vi "Chain4.vi"(7 "Name (\"\" to Use UUID)":string="CSM-Module") -> ()   [LabVIEW 2017, in "CSM-Testcase.lvlib"]
doc: "Creates a template for a CSM module without a user interface.\n\n> [!NOTE] CSM Name Rules\n> - The CSM module name must be unique to avoid entering the \"Critical Error\" state.\n> - If the input is \"\", a UUID will be used as the module name. This module will operate in independent mode and will not be listed in the module list.\n> - If the input ends with '#', the module will run in work mode. Modules with the same name will share the same message queue. External messages will be handled by the idle module.\n\n> [!NOTE] CSM Initialization State\n> - The default value is \"Macro: Initialize\", consistent with the JKISM state machine.\n> - This state is typically not modified and is provided to facilitate external programmatic changes to the initialization state.\n\n\n-- <b>Controls</b> --\n- <b>Name (\"\" to Use UUID)</b>: CSM Module Name\n- <b>Init State(\"Macro: Initialize\")</b>: Initialization State, default is \"Macro: Initialize\""
uses:
  CSM-Testcase.lvlib
  src/user.lib/_NEVSTOP/Communicable State Machine(CSM)/AdvanceAPI/CSM - Revert Arguments-Safe String.vi
  src/user.lib/_NEVSTOP/Communicable State Machine(CSM)/AdvanceAPI/CSM - Make String Arguments Safe.vi
  src/user.lib/_NEVSTOP/Communicable State Machine(CSM)/AdvanceAPI/CSM - Break Down Multiple States String.vi
  src/user.lib/_NEVSTOP/Communicable State Machine(CSM)/AdvanceAPI/CSM - Keywords.vi
  src/user.lib/_NEVSTOP/Communicable State Machine(CSM)/_Shared/Trim Single-line Text.vi
  Global-TestcaseCSM.vi
  src/user.lib/_NEVSTOP/Communicable State Machine(CSM)/_Polymophic/Build No-Reply Asynchronous Message with Arguments.vi
  src/user.lib/_NEVSTOP/Communicable State Machine(CSM)/_Polymophic/Build Asynchronous Message with Arguments.vi
  src/user.lib/_NEVSTOP/Communicable State Machine(CSM)/_Polymophic/Build Register Message.vi
  src/user.lib/_NEVSTOP/Communicable State Machine(CSM)/_Polymophic/Build Interrupt Broadcast Message.vi
  src/user.lib/_NEVSTOP/Communicable State Machine(CSM)/Communicable State Machine.lvlib
panel:
  out "Error Occurred":errorcluster
  out "State History":string
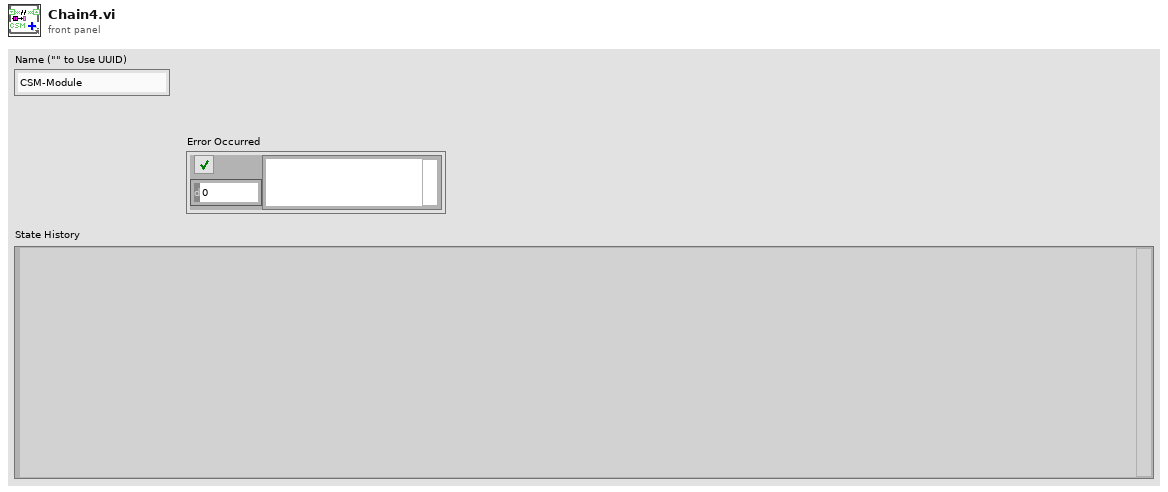
[diagram p1: front panel]
types:
  T1 = cluster{"Arguments":string, "Response":string, "error":errorcluster}
  T2 = enum32{"Invalid", "Standard", "Closed", "Hidden", "Minimized", "Maximized"}
  T3 = enum32{"invalid app kind", "Development System", "Run Time System", "Student Edition", "Embedded LabVIEW", "Evaluation", "Custom"}
  T4 = typedef "Communicable State Machine.lvlib/_CSM_Response Source Message.ctl" = cluster{"‘State":string, "’Arguments":string, "’Error":errorcluster}
  T5 = cluster{"Current VI Reference":refnum<vi>, "Close Panel on Exit?":bool}
  T6 = cluster{"Core":cluster{"Current VI Reference":refnum<vi>, "Close Panel on Exit?":bool}, "Your Boolean data":bool, "Your string data":string, "Counter":u32}
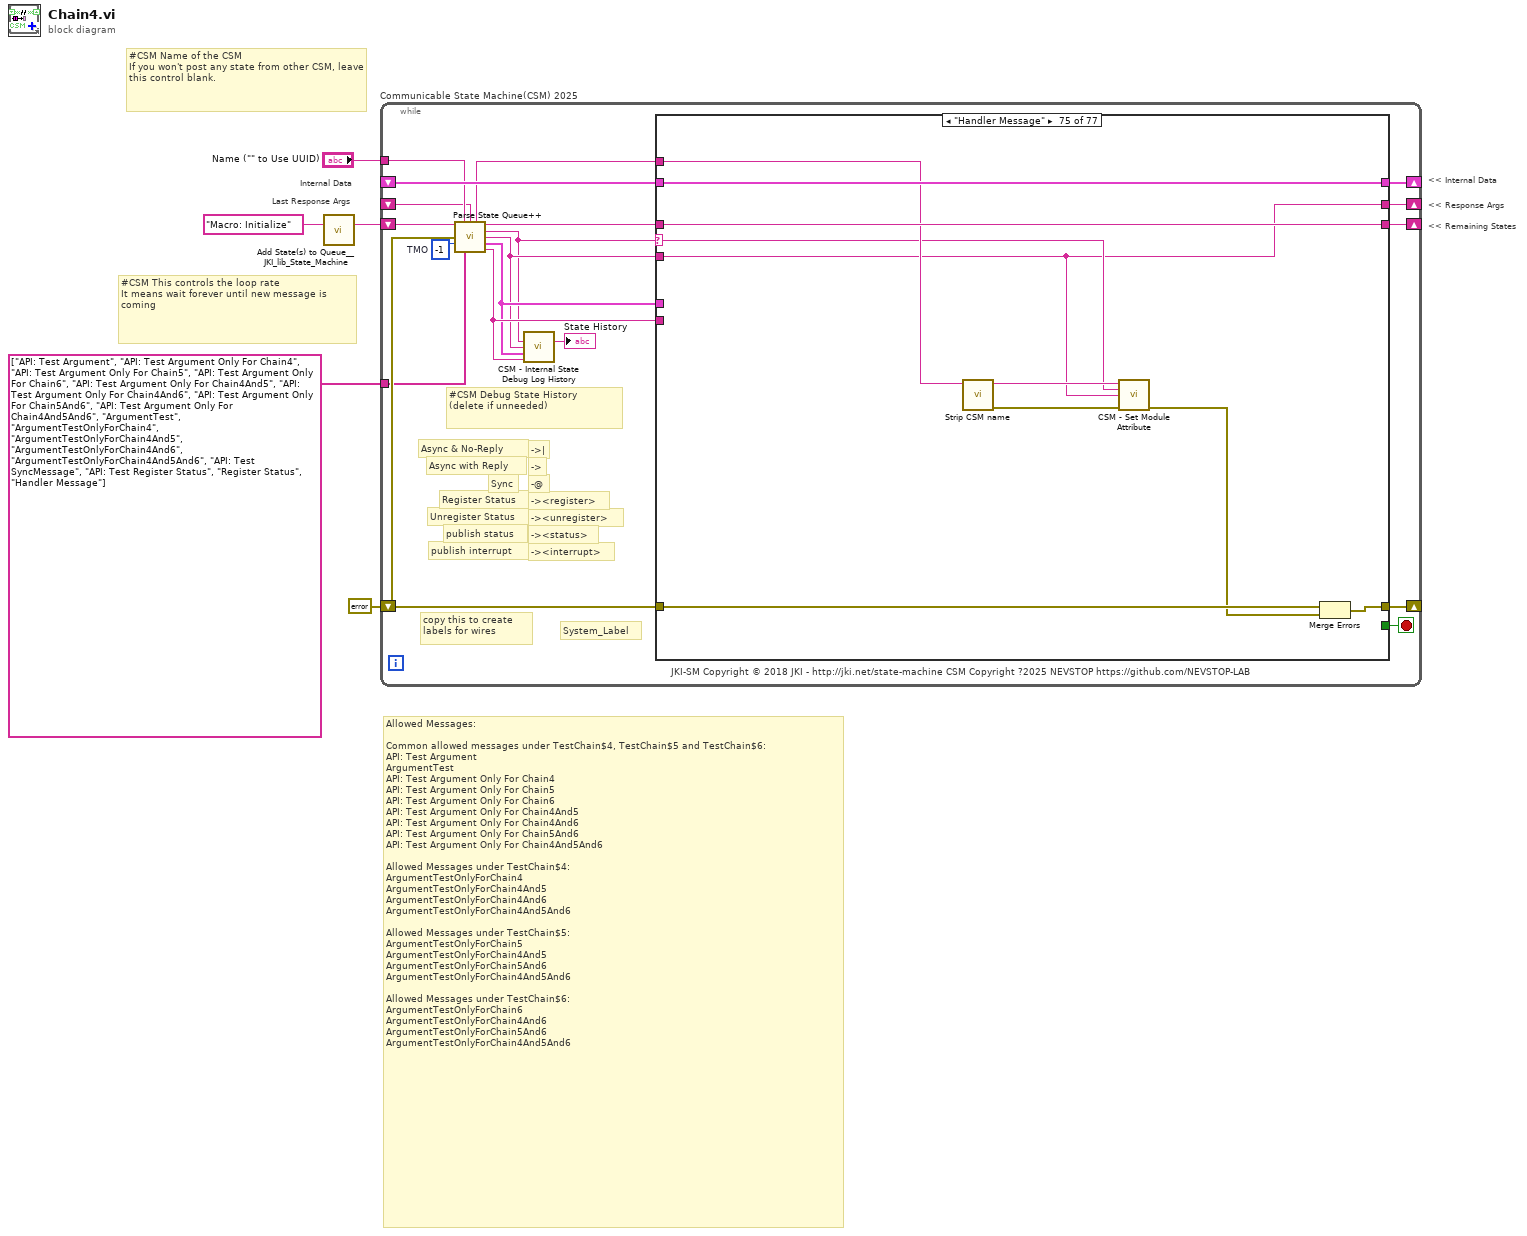
[diagram p0: block diagram]
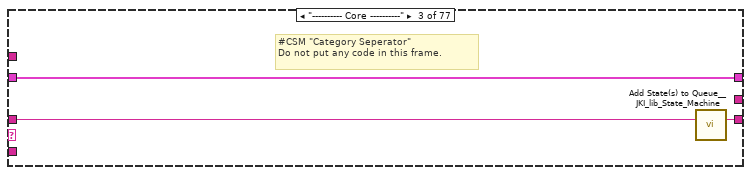
[diagram p4: hidden frame]
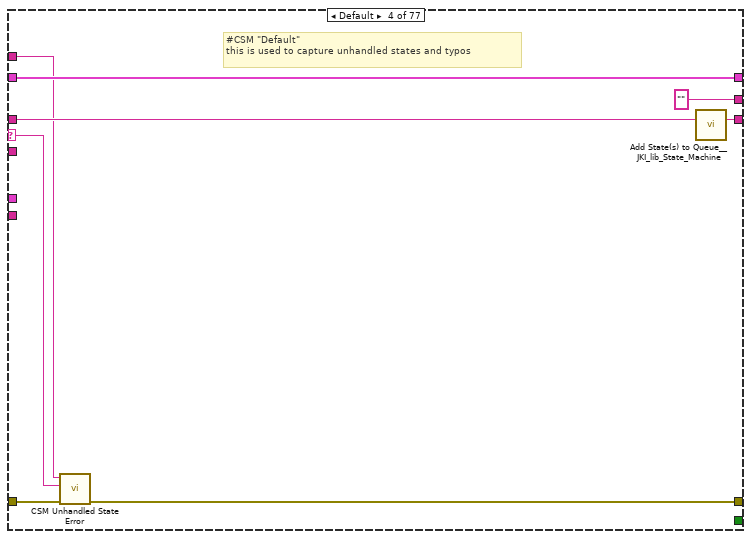
[diagram p5: hidden frame]
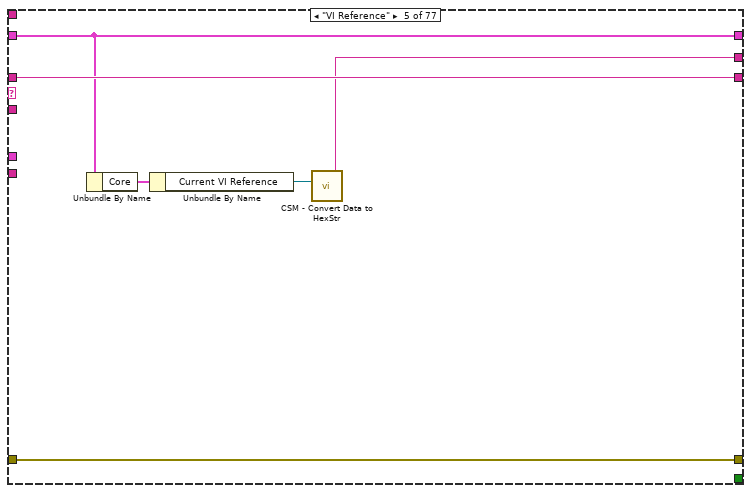
[diagram p6: hidden frame]
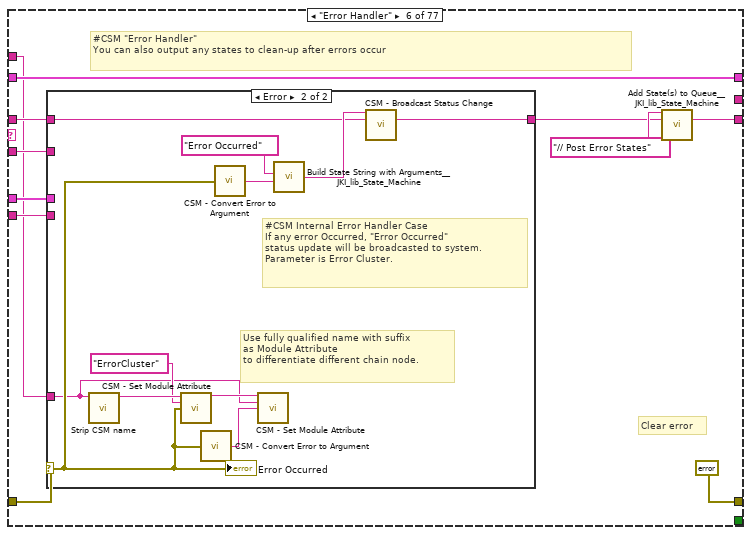
[diagram p7: hidden frame]
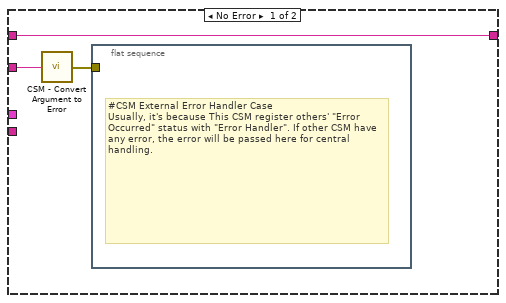
[diagram p8: hidden frame]
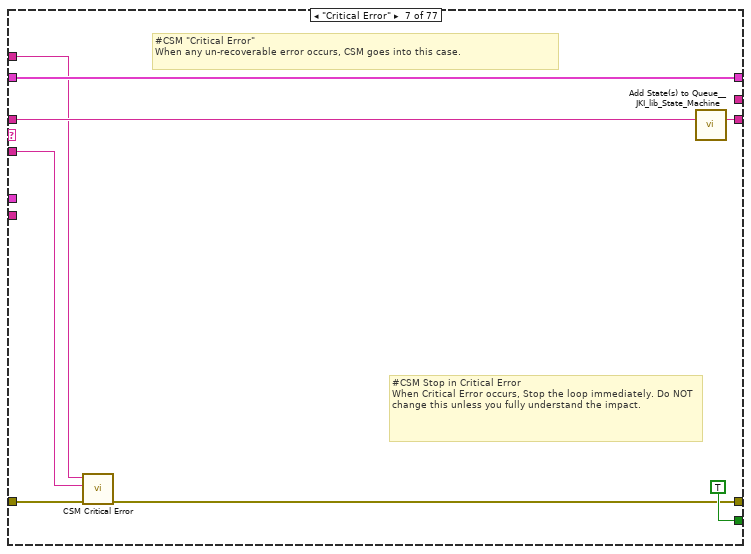
[diagram p9: hidden frame]
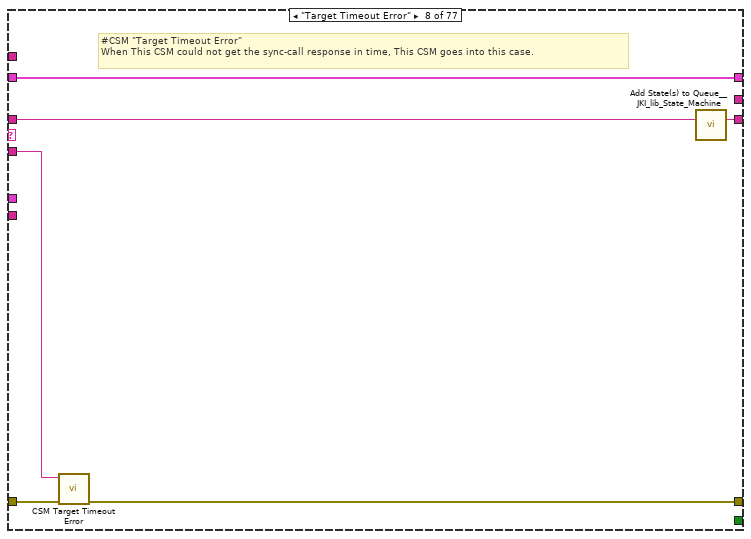
[diagram p10: hidden frame]
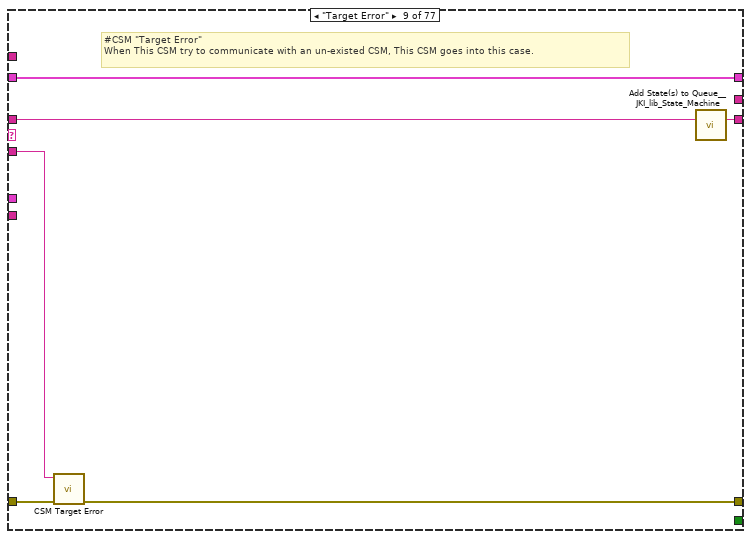
[diagram p11: hidden frame]
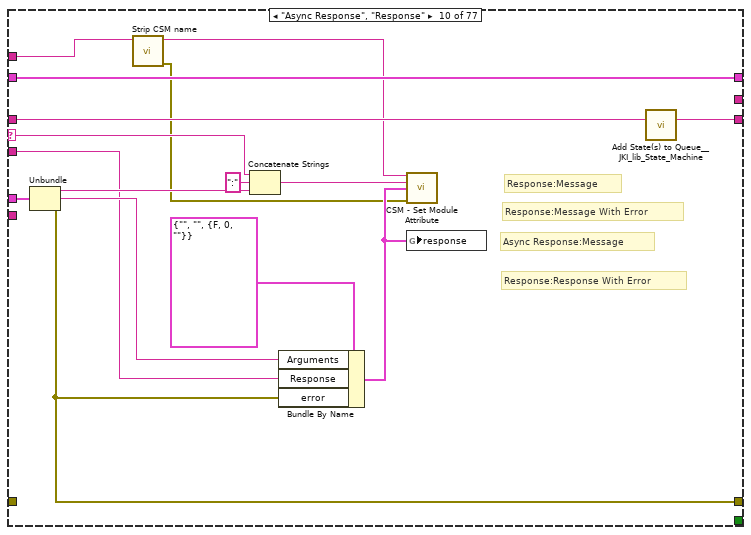
[diagram p12: hidden frame]
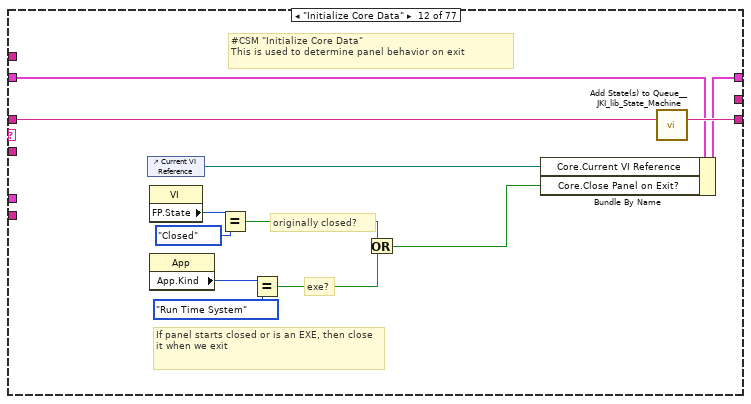
[diagram p14: hidden frame]
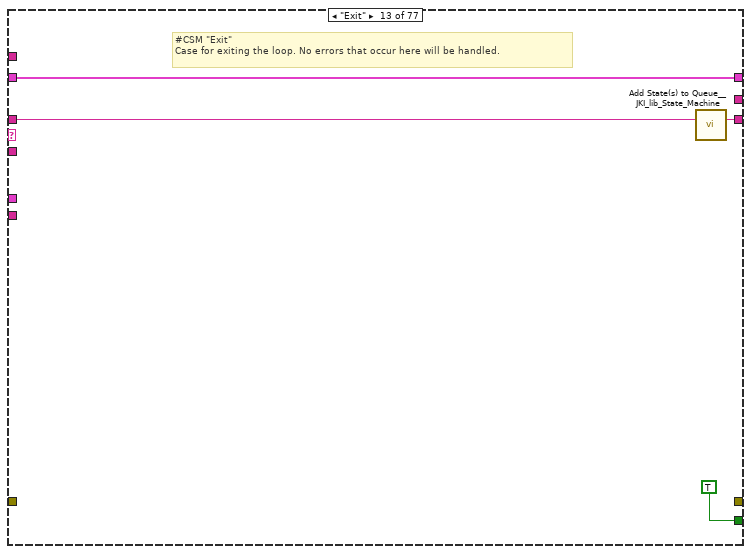
[diagram p15: hidden frame]
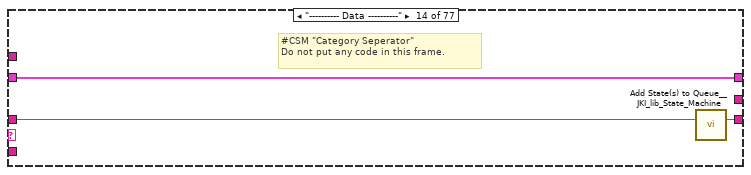
[diagram p16: hidden frame]
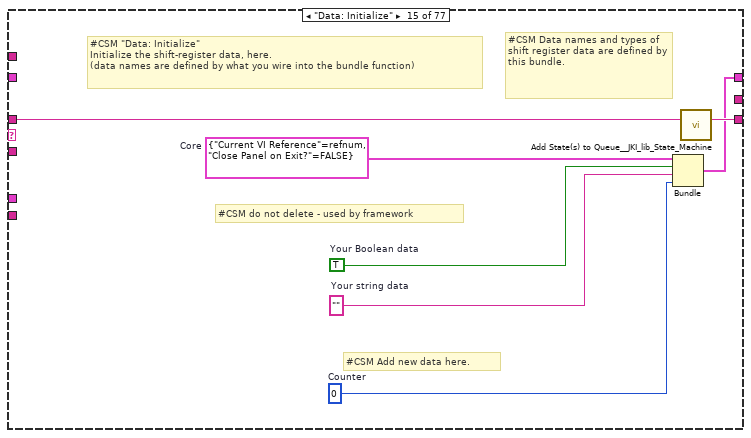
[diagram p17: hidden frame]
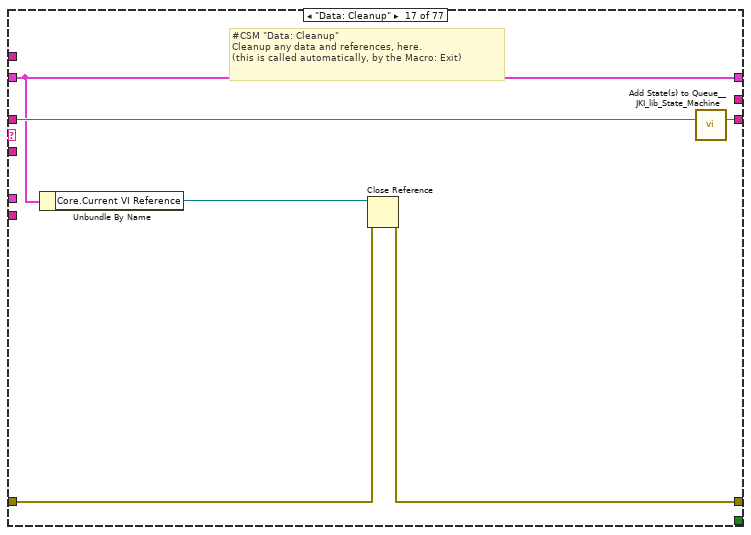
[diagram p19: hidden frame]
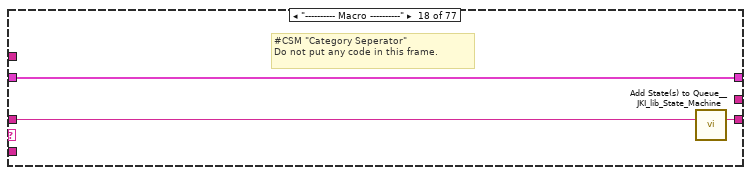
[diagram p20: hidden frame]
diagram:
  # "Allowed Messages:\n\nCommon allowed messages under TestChain$4, TestChain$5 and TestChain$6:\nAPI: Test Argument\nArgumentTest\nAPI: Test Argument Only For Chain4\nAPI: Test Argument Only For Chain5\nAPI: Test Argument Only For Chain6\nAPI: Test Argument Only For Chain4And5\nAPI: Test Argument Only For Chain4And6\nAPI: Test Argument Only For Chain5And6\nAPI: Test Argument Only For Chain4And5And6\n\nAllowed Messages under TestChain$4:\nArgumentTestOnlyForChain4\nArgumentTestOnlyForChain4And5\nArgumentTestOnlyForChain4And6\nArgumentTestOnlyForChain4And5And6\n\nAllowed Messages under TestChain$5:\nArgumentTestOnlyForChain5\nArgumentTestOnlyForChain4And5\nArgumentTestOnlyForChain5And6\nArgumentTestOnlyForChain4And5And6\n\nAllowed Messages under TestChain$6:\nArgumentTestOnlyForChain6\nArgumentTestOnlyForChain4And6\nArgumentTestOnlyForChain5And6\nArgumentTestOnlyForChain4And5And6"
  # "Last Response Args"
  # "Internal Data"
  # "#CSM Name of the CSM\nIf you won't post any state from other CSM, leave this control blank."
  # "#CSM This controls the loop rate\nIt means wait forever until new message is coming"
  # "<< Internal Data"
  # "<< Response Args"
  # "<< Remaining States"
  n1 = call <vilib>:"Add State(s) to Queue__JKI_lib_State_Machine.vi"("State(s) in (\"\")"="Macro: Initialize" ("Init State(\"Macro: Initialize\")")) -> ("States Out"=w5:string)  [unwired: 14 in]
  n2 = while "Communicable State Machine(CSM) 2025" {
    shift-right: [w19] -> _
    shift-left: _ -> [w18]
    shift-right: [w22] -> _
    shift-left: errorcluster {"status"=FALSE, "code"=0, "source"=""} ("error out") -> [w8]
    shift-right: [w21] -> _
    shift-left: w5 -> [w23]
    tunnel: "Name (\"\" to Use UUID)" -> [w15]
    shift-right: [w16] -> _
    shift-left: _ -> [w10]
    tunnel: string[] ["API: Test Argument", "API: Test Argument Only For Chain4", "API: Test Argument Only For Chain5", "API: Test Argument Only For Chain6", "API: Test Argument Only For Chain4And5", "API: Test Argument Only For Chain4And6", "API: Test Argument Only For Chain5And6", "API: Test Argument Only For Chain4And5And6", "ArgumentTest", "ArgumentTestOnlyForChain4", "ArgumentTestOnlyForChain4And5", "ArgumentTestOnlyForChain4And6", "ArgumentTestOnlyForChain4And5And6", "API: Test SyncMessage", "API: Test Register Status", "Register Status", "Handler Message"] ("Allowed Messages (Empty for All)") -> [w6]
    stop <- w20 stop-if-true
    w17 = -1  # TMO
    # "#CSM Debug State History\n(delete if unneeded)"
    # "-><interrupt>"
    # "-><status>"
    # "-><unregister>"
    # "-><register>"
    # "-@"
    # "->"
    # "->|"
    # "publish interrupt"
    # "publish status"
    # "Unregister Status"
    # "Register Status"
    # "Sync"
    # "Async with Reply"
    # "Async & No-Reply"
    # "JKI-SM Copyright © 2018 JKI - http://jki.net/state-machine CSM Copyright ?2025 NEVSTOP https://github.com/NEVSTOP-LAB"
    # "copy this to create labels for wires"
    # "System_Label"
    n3 = call "Parse State Queue++.vi"("State Queue"=w23, "Name (\"\" to Use UUID)"=w15, "Response Arguments"=w10, "Previous Error"=w8, "Dequeue (1 ms)"=w17, "Allowed Messages (Empty for All)"=w6) -> ("Name Used"=w9:string, "Remaining States"=w24:string, "Current State"=w11:string, "Arguments"=w12:string, "Additional Information"=w13:T4, "Source CSM"=w14:string)  [unwired: 4 in]
    n4 = call "CSM - Internal State Debug Log History.vi"("State"=w11, "Arguments (\"\")"=w12, ">> Response Source Message >>"=w13, "Source (\"\")"=w14) -> ("Debug Log"=→"State History":string)  [unwired: 11 in]
    n5 = case shown="\"Handler Message\"" w11 {
      selector: w11 -> [_ _ _ w35 _ _ _ _ _ w102 _ _ _ _ _ _ _ _ _ _ _ _ _ _ _ _ _ _ _ _ _ _ _ w389 _ _ _ _ _ _ _ _ _ _ _ _ _ _ _ _ _ _ _ _ _ _ w581 _ _ _ _ _ _ _ _ _ _ w649 _ _ _ w674 _ w696 w703 w719 _]
      tunnel: w24 -> [w25 w28 w31 w39 w44 w50 w78 w84 w90 w106 w108 w120 w124 w127 w134 w136 w142 w145 w149 w155 w169 w189 w218 w222 w226 w238 w266 w298 w314 w326 w338 w352 w375 w407 w423 w436 w443 w450 w457 w464 w471 w478 w485 w492 w499 w506 w513 w525 w534 w544 w554 w564 w568 w573 w576 w580 w587 w594 w597 w610 w616 w622 w626 w631 w635 w639 w643 w653 w657 w665 w671 w679 w689 w698 w708 w724 w736]
      tunnel: w12 -> [_ _ _ _ _ w49 w74 w81 w87 w96 _ _ _ _ _ _ _ _ _ _ w156 w176 w201 _ w229 w241 w269 w301 w317 w329 w341 w355 w371 w405 w426 w433 w440 w447 w454 w461 w468 w475 w482 w489 w496 w503 w510 w517 _ w536 w545 w555 w566 _ _ w577 _ w590 w599 _ w612 w618 w624 w629 w634 w638 w642 w648 w656 w663 w669 w676 w685 w697 w702 w714 _]
      tunnel: w18 -> [w26 w27 w29 w37 w43 w55 w76 w82 w88 w104 w107 w114 w122 w125 _ w135 w137 w143 w147 w153 w171 w191 w220 w221 w230 w242 w270 w302 w318 w330 w342 w356 w378 w410 w427 w438 w445 w452 w459 w466 w473 w480 w487 w494 w501 w508 w515 w523 w532 w542 w552 w562 w567 w571 w574 w578 w588 w595 w601 w611 w617 w623 w628 w633 w636 w640 w644 w654 w658 w664 w670 w680 w683 w699 w709 w716 w734]
      tunnel: [_ _ _ w32 w45 errorcluster {"status"=FALSE, "code"=0, "source"=""} ("error out") w71 w79 w85 w95 _ _ _ _ _ _ w138 _ _ _ _ _ _ _ w223 w235 w263 w295 w311 w323 w335 w348 w372 w391 w420 w437 w444 w451 w458 w465 w472 w479 w486 w493 w500 w507 w514 w519 w528 w538 w549 w559 _ _ _ _ w583 _ _ w603 _ _ w627 w632 w637 w641 w645 w647 w659 w660 w666 w673 w686 w692 w704 w720 _] -> w22
      tunnel: w8 -> [_ _ _ w33 w45 w53 w72 w80 w86 _ _ _ _ _ _ _ w139 _ _ _ _ _ _ _ _ _ _ _ _ _ _ _ _ _ _ w437 w444 w451 w458 w465 w472 w479 w486 w493 w500 w507 w514 _ _ _ _ _ _ _ _ _ _ _ _ _ _ _ w627 w632 w637 w641 w645 w655 w659 w661 w667 w681 w690 w700 w710 w725 _]
      tunnel: [w25 w28 w30 w38 w44 w51 w77 w83 w89 w105 w108 w119 w123 w126 w133 w136 w141 w144 w148 w154 w170 w190 w219 w222 w227 w239 w267 w299 w315 w327 w339 w353 w376 w408 w424 w435 w442 w449 w456 w463 w470 w477 w484 w491 w498 w505 w512 w524 w533 w543 w553 w563 w568 w572 w575 w579 w589 w591 w596 w608 w613 w619 w625 w630 w635 w639 w643 w653 w657 w665 w671 w679 w689 w698 w708 w724 w735] -> w21
      tunnel: [_ _ _ _ _ _ TRUE _ _ _ _ _ TRUE _ _ _ _ _ _ _ _ _ _ _ _ _ _ _ _ _ _ _ _ _ _ _ _ _ _ _ _ _ _ _ _ _ _ _ _ _ _ _ _ _ _ _ _ _ _ _ _ _ _ _ _ _ _ _ _ _ _ _ _ _ _ _ _] -> w20
      tunnel: [w26 w27 w29 w37 w43 w55 w76 w82 w88 w104 w107 w118 w122 w125 w132 w135 w137 w143 w147 w153 w171 w191 w220 w221 w230 w242 w270 w302 w318 w330 w342 w356 w378 w410 w427 w438 w445 w452 w459 w466 w473 w480 w487 w494 w501 w508 w515 w523 w532 w542 w552 w562 w567 w571 w574 w578 w588 w595 w601 w611 w617 w623 w628 w633 w636 w640 w644 w654 w658 w664 w670 w680 w683 w699 w709 w715 w732] -> w19
      tunnel: w14 -> [_ _ _ _ _ w48 _ _ _ _ _ _ _ _ _ _ _ _ _ _ _ _ _ _ _ _ _ _ _ _ _ _ _ _ _ _ _ _ _ _ _ _ _ _ _ _ _ _ _ _ _ _ _ _ _ _ _ _ _ _ _ _ _ _ _ _ _ _ _ _ _ _ _ _ _ _ _]
      tunnel: w13 -> [_ _ _ _ _ w47 _ _ _ w103 _ _ _ _ _ _ _ _ _ _ _ _ _ _ _ _ _ _ _ _ _ _ _ _ _ _ _ _ _ _ _ _ _ _ _ _ _ _ _ _ _ _ _ _ _ _ _ _ _ _ _ _ _ _ _ _ _ _ _ _ _ _ _ _ _ _ _]
      tunnel: [_ _ _ "" w40 _ _ _ _ _ _ _ _ _ _ _ _ _ _ _ _ _ _ _ _ _ _ _ _ _ _ _ _ w392 _ _ _ _ _ _ _ _ _ _ _ _ _ _ _ _ _ _ w565 _ _ w577 w582 _ _ _ _ _ w624 w629 w634 w638 w642 w648 w656 w663 w669 _ w685 w697 w702 _ _] -> w16
      tunnel: w9 -> [_ _ _ w34 _ w46 w73 _ _ w93 _ _ _ _ _ _ _ _ _ _ _ _ _ _ _ _ w254 w286 _ _ _ w349 _ w395 _ _ _ _ _ _ _ _ _ _ _ _ _ w521 w530 w540 w551 w561 _ _ _ _ w584 _ _ w605 _ _ _ _ _ _ _ w652 _ _ _ w678 w682 w695 w707 w723 _]
      frame "", "Idle" {
        # "#CSM \"Idle/Event Handler\"\nexecutes when the state queue is empty"
      }
      frame "CSM Documentation" {
        # "#CSM State Syntax\n\n// Comment line, all text to the right of “//” will be ignored\n// Local Message Example\nDoSth: DoA >> Arguments\n\n// Sync Call Example\nAPI: xxxx >> Arguments -@ TargetModule\n\n// Async Call Example\nAPI: xxxx >> Arguments -> TargetModule\n\n// Async Call without Reply Example\nAPI: xxxx >> Arguments ->| TargetModule\n\n// Broadcast normal status:\nStatus >> StatusArguments  -><status>\n\n// Broadcast Interrupt status:\nInterrupt >> StatusArguments  -><interrupt>\n\n// Register Source Module's status to Handler Module\nStatus@Source Module >> Handler Module@Handler Module -><register>\n\n// Unegister Source Module's status\nStatus@Source Module >> Handler Module -><unregister>"
        # "#CSM README FIRST\n\nCommunicable State Machine(CSM) is a LabVIEW application framework that builds upon JKI State Machine(JKISM). It follows the pattern of JKISM and extends the keywords to describe message communication between modules, including concepts such as Sync-Message, Async-Message, Subscription/Unsubscription of status - essential elements for creating reusable code modules. For more information, please visit the CSM wiki: https://nevstop-lab.github.io/CSM-Wiki/\n\nFor instructions on JKI State Machine, visit: \n    http://jki.net/state-machine/\nFor information about CSM, visit: \n    https://github.com/NEVSTOP-LAB"
        # "#CSM \"Documentation\"\nCase for holding CSM Documenation"
      }
      frame "---------- Core ----------" {
        # "#CSM \"Category Seperator\"\nDo not put any code in this frame."
        n6 = call <vilib>:"Add State(s) to Queue__JKI_lib_State_Machine.vi"("State(s) in (\"\")"=w31) -> ("States Out"=w30:string)  [unwired: 14 in]
      }
      frame Default {
        # "#CSM \"Default\"\nthis is used to capture unhandled states and typos"
        n7 = call "CSM Unhandled State Error.vi"("error in (no error)"=w33, "Undefined State"=w35, "CSM Name"=w34) -> ("error out"=w32:errorcluster)  [unwired: 8 in]
        n8 = call <vilib>:"Add State(s) to Queue__JKI_lib_State_Machine.vi"("State(s) in (\"\")"=w39) -> ("States Out"=w38:string)  [unwired: 14 in]
      }
      frame "VI Reference" {
        n9 = Unbundle By Name(w43) -> ("Core"=w42:T5)
        n10 = Unbundle By Name(w42) -> ("Current VI Reference"=w41:refnum<vi>)
        n11 = call "CSM - Convert Data to HexStr.vi"("Variant"=w41) -> ("HEX String (0-9,A-F)"=w40:string)  [unwired: 8 in]
      }
      frame "Error Handler" {
        # "#CSM \"Error Handler\"\nYou can also output any states to clean-up after errors occur"
        # "Clear error"
        n12 = case shown="Error" w53 {
          selector: w53 -> [_ w62]
          tunnel: [w59 w67] -> w52
          tunnel: w50 -> [w59 w66]
          tunnel: w49 -> [w58 _]
          tunnel: w48 -> [_ _]
          tunnel: w47 -> [_ _]
          tunnel: w46 -> [_ w60]
          frame No Error {
            n13 = call "CSM - Convert Argument to Error.vi"("Argument"=w58) -> ("Error"=w57:errorcluster)  [unwired: 4 in]
            n14 = flat-sequence {
              tunnel: w57 -> [_]
              frame #0 {
                # "#CSM External Error Handler Case\nUsually, it's because This CSM register others' \"Error Occurred\" status with \"Error Handler\". If other CSM have any error, the error will be passed here for central handling."
              }
            }
          }
          frame Error {
            # "Use fully qualified name with suffix \nas Module Attribute  \nto differentiate different chain node."
            # "#CSM Internal Error Handler Case \nIf any error Occurred, \"Error Occurred\" \nstatus update will be broadcasted to system.\nParameter is Error Cluster."
            n15 = call "Strip CSM name.vi"("CSM name"=w60) -> ("CSM name core"=w65:string)  [unwired: 7 in, 3 out]
            n16 = call "CSM - Set Module Attribute.vi"("CSM Name"=w65, "Attribute"="ErrorCluster", "Value"=w62) -> ("CSM Name (Dup)"=w63:string)  [unwired: 9 in, 3 out]
            n17 = call "CSM - Convert Error to Argument.vi"("Error"=w62) -> ("Argument"=w61:string)  [unwired: 4 in]
            n18 = call "CSM - Convert Error to Argument.vi"("Error"=w62) -> ("Argument"=w69:string)  [unwired: 4 in]
            n19 = call "CSM - Set Module Attribute.vi"("CSM Name"=w63, "Attribute"=w60, "Value"=w61) -> ()  [unwired: 9 in, 4 out]
            n20 = call <vilib>:"Build State String with Arguments__JKI_lib_State_Machine.vi"("Arguments (\"\")"=w69, "State"="Error Occurred" ("Status with Arguments")) -> ("State with Arguments"=w68:string)  [unwired: 4 in]
            n21 = call "CSM - Broadcast Status Change.vi"("Status With Arguments"=w68, "State Queue"=w66) -> ("Remaining States"=w67:string)  [unwired: 13 in]
            "Error Occurred" <- w62
          }
        }
        n22 = call <vilib>:"Add State(s) to Queue__JKI_lib_State_Machine.vi"("State(s) in Front (\"\")"="// Post Error States", "State(s) in (\"\")"=w52) -> ("States Out"=w51:string)  [unwired: 13 in]
      }
      frame "Critical Error" {
        # "#CSM \"Critical Error\"\nWhen any un-recoverable error occurs, CSM goes into this case."
        # "#CSM Stop in Critical Error\nWhen Critical Error occurs, Stop the loop immediately. Do NOT change this unless you fully understand the impact."
        n23 = call "CSM Critical Error.vi"("error in (no error)"=w72, "Arugments (As Reason)"=w74, "CSM Name"=w73) -> ("error out"=w71:errorcluster)  [unwired: 8 in]
        n24 = call <vilib>:"Add State(s) to Queue__JKI_lib_State_Machine.vi"("State(s) in (\"\")"=w78) -> ("States Out"=w77:string)  [unwired: 14 in]
      }
      frame "Target Timeout Error" {
        # "#CSM \"Target Timeout Error\"\nWhen This CSM could not get the sync-call response in time, This CSM goes into this case."
        n25 = call "CSM Target Timeout Error.vi"("error in (no error)"=w80, "Arguments (As CSM Name)"=w81) -> ("error out"=w79:errorcluster)  [unwired: 9 in]
        n26 = call <vilib>:"Add State(s) to Queue__JKI_lib_State_Machine.vi"("State(s) in (\"\")"=w84) -> ("States Out"=w83:string)  [unwired: 14 in]
      }
      frame "Target Error" {
        # "#CSM \"Target Error\"\nWhen This CSM try to communicate with an un-existed CSM, This CSM goes into this case."
        n27 = call "CSM Target Error.vi"("error in (no error)"=w86, "Arguments (As CSM Name)"=w87) -> ("error out"=w85:errorcluster)  [unwired: 9 in]
        n28 = call <vilib>:"Add State(s) to Queue__JKI_lib_State_Machine.vi"("State(s) in (\"\")"=w90) -> ("States Out"=w89:string)  [unwired: 14 in]
      }
      frame "Async Response", "Response" {
        # "Response:Response With Error"
        # "Response:Message With Error"
        # "Async Response:Message"
        # "Response:Message"
        n29 = Unbundle(w103) -> ("‘State"=w101:string, "’Arguments"=w97:string, "’Error"=w95:errorcluster)
        n30 = call "Strip CSM name.vi"("CSM name"=w93) -> ("error out"=w91:errorcluster, "CSM name core"=w92:string)  [unwired: 7 in, 2 out]
        n31 = Concatenate Strings(w102, ":" ("string"), w101) -> (w99:string)
        n32 = Bundle By Name(cluster=T1 {"Arguments"="", "Response"="", "error"={"status"=FALSE, "code"=0, "source"=""}}, "Arguments"=w97, "Response"=w96, "error"=w95) -> (w94:T1)
        n33 = call "CSM - Set Module Attribute.vi"("CSM Name"=w92, "Attribute"=w99, "Value"=w94, "Error In"=w91) -> ()  [unwired: 8 in, 4 out]
        n34 = global write "Global-TestcaseCSM.vi" "response"(w94) -> ()
        n35 = call <vilib>:"Add State(s) to Queue__JKI_lib_State_Machine.vi"("State(s) in (\"\")"=w106) -> ("States Out"=w105:string)  [unwired: 14 in]
      }
      frame "Async Message Posted" {
        # "#CSM \"Async Message Posted\"\nAfter Async Message is posted (-> or ->| ), CSM goes to this state for post-action.\nYou can use Argument - State to tell which Async Message is called."
      }
      frame "Initialize Core Data" {
        # "#CSM \"Initialize Core Data\"\nThis is used to determine panel behavior on exit"
        # "originally closed?"
        # "exe?"
        # "If panel starts closed or is an EXE, then close it when we exit"
        n36 = control-ref of="Current VI Reference"() -> (w112:refnum<vi>)
        n37 = property class="VI"() -> ("FP.State"=w111:T2)  [unwired: 2 in, 2 out]
        n38 = property class="App"() -> ("App.Kind"=w117:T3)  [unwired: 2 in, 2 out]
        n39 = Equal?(x=w111, y=T2."Closed" ("Front Panel Window:State")) -> (x = y?=w109:bool)
        n40 = Equal?(x=w117, y=T3."Run Time System" ("Application:Kind")) -> (x = y?=w115:bool)
        n41 = Or(x=w109, y=w115) -> (x .or. y?=w113:bool)
        n42 = Bundle By Name(cluster=w114, "Core.Current VI Reference"=w112, "Core.Close Panel on Exit?"=w113) -> (w118:T6)
        n43 = call <vilib>:"Add State(s) to Queue__JKI_lib_State_Machine.vi"("State(s) in (\"\")"=w120) -> ("States Out"=w119:string)  [unwired: 14 in]
      }
      frame "Exit" {
        # "#CSM \"Exit\"\nCase for exiting the loop. No errors that occur here will be handled."
        n44 = call <vilib>:"Add State(s) to Queue__JKI_lib_State_Machine.vi"("State(s) in (\"\")"=w124) -> ("States Out"=w123:string)  [unwired: 14 in]
      }
      frame "---------- Data ----------" {
        # "#CSM \"Category Seperator\"\nDo not put any code in this frame."
        n45 = call <vilib>:"Add State(s) to Queue__JKI_lib_State_Machine.vi"("State(s) in (\"\")"=w127) -> ("States Out"=w126:string)  [unwired: 14 in]
      }
      frame "Data: Initialize" {
        w128 = u32 0  # Counter
        w129 = T5 {"Current VI Reference"=refnum, "Close Panel on Exit?"=FALSE}  # Core
        w131 = TRUE  # Your Boolean data
        w130 = ""  # Your string data
        # "#CSM \"Data: Initialize\"\nInitialize the shift-register data, here.\n(data names are defined by what you wire into the bundle function)"
        # "#CSM do not delete - used by framework"
        # "#CSM Add new data here."
        # "#CSM Data names and types of shift register data are defined by this bundle."
        n46 = Bundle("Core"=w129, "Your Boolean data"=w131, "Your string data"=w130, "Counter"=w128) -> (w132:T6)  [unwired: 1 in]
        n47 = call <vilib>:"Add State(s) to Queue__JKI_lib_State_Machine.vi"("State(s) in (\"\")"=w134) -> ("States Out"=w133:string)  [unwired: 14 in]
      }
      frame "Data: Update Indicators" {
      }
      frame "Data: Cleanup" {
        # "#CSM \"Data: Cleanup\"\nCleanup any data and references, here.\n(this is called automatically, by the Macro: Exit)"
        n48 = Unbundle By Name(w137) -> ("Core.Current VI Reference"=w140:refnum<vi>)
        n49 = Close Reference(reference=w140, error in (no error)=w139) -> (error out=w138:errorcluster)
        n50 = call <vilib>:"Add State(s) to Queue__JKI_lib_State_Machine.vi"("State(s) in (\"\")"=w142) -> ("States Out"=w141:string)  [unwired: 14 in]
      }
      frame "---------- Macro ----------" {
        # "#CSM \"Category Seperator\"\nDo not put any code in this frame."
        n51 = call <vilib>:"Add State(s) to Queue__JKI_lib_State_Machine.vi"("State(s) in (\"\")"=w145) -> ("States Out"=w144:string)  [unwired: 14 in]
      }
      frame "Macro: Initialize" {
        # "#CSM \"Macro: Initialize\"\nInitialization Macro (This is called once, when the VI starts)"
        n52 = call <vilib>:"Add State(s) to Queue__JKI_lib_State_Machine.vi"("State(s) in Front (\"\")"="Data: Initialize\nInitialize Core Data\nData: Update Indicators", "State(s) in (\"\")"=w149) -> ("States Out"=w148:string)  [unwired: 13 in]
      }
      frame "Macro: Exit" {
        # "#CSM \"Macro: Exit\"\nExit Macro (This is called once, when the VI exits)"
        n53 = call <vilib>:"Add State(s) to Queue__JKI_lib_State_Machine.vi"("State(s) in Front (\"\")"="//Exit Sub-Modules ", "State(s) at Back (\"\")"="Data: Cleanup\nExit") -> ("States Out"=w151:string)  [unwired: 13 in]
        n54 = call <vilib>:"Add State(s) to Queue__JKI_lib_State_Machine.vi"("State(s) in Front (\"\")"=w151, "State(s) in (\"\")"=w155) -> ("States Out"=w154:string)  [unwired: 13 in]
      }
      frame "Macro: Test MacroWithSubMessages" {
        w157 = "SubMessage2" ("State With Arguments")
        w159 = "SubMessage1" ("State With Arguments")
        n55 = call "uuid.vi"() -> ("UUID"=w158:string)  [unwired: 11 in]
        n56 = call "uuid.vi"() -> ("UUID"=w160:string)  [unwired: 11 in]
        n57 = Concatenate Strings(w159, w160) -> (w161:string)
        n58 = Concatenate Strings(w157, w158) -> (w162:string)
        n59 = call <vilib>:"Build State String with Arguments__JKI_lib_State_Machine.vi"("Arguments (\"\")"=w156, "State"="SubMessage3" ("State With Arguments")) -> ("State with Arguments"=w164:string)  [unwired: 4 in]
        n60 = call <vilib>:"Build State String with Arguments__JKI_lib_State_Machine.vi"("Arguments (\"\")"=w161, "State"=w159) -> ("State with Arguments"=w166:string)  [unwired: 4 in]
        n61 = call <vilib>:"Build State String with Arguments__JKI_lib_State_Machine.vi"("Arguments (\"\")"=w162, "State"=w157) -> ("State with Arguments"=w165:string)  [unwired: 4 in]
        n62 = Build Array(w166, w165, w164) -> (w163:string[])
        n63 = call "CSM - Compact Multiple States.vi"("Multiple States"=w163) -> ("States"=w168:string)  [unwired: 9 in]
        n64 = call <vilib>:"Add State(s) to Queue__JKI_lib_State_Machine.vi"("State(s) in Front (\"\")"=w168, "State(s) in (\"\")"=w169) -> ("States Out"=w170:string)  [unwired: 13 in]
      }
      frame "Macro: Test MacroWithSubAndPostMessages" {
        w175 = "PostMessage1" ("State With Arguments")
        w177 = "SubMessage2" ("State With Arguments")
        w179 = "SubMessage1" ("State With Arguments")
        n65 = call "uuid.vi"() -> ("UUID"=w178:string)  [unwired: 11 in]
        n66 = call "uuid.vi"() -> ("UUID"=w174:string)  [unwired: 11 in]
        n67 = call "uuid.vi"() -> ("UUID"=w180:string)  [unwired: 11 in]
        n68 = Concatenate Strings(w175, w174) -> (w173:string)
        n69 = Concatenate Strings(w179, w180) -> (w181:string)
        n70 = Concatenate Strings(w177, w178) -> (w182:string)
        n71 = call <vilib>:"Build State String with Arguments__JKI_lib_State_Machine.vi"("Arguments (\"\")"=w176, "State"="SubMessage3" ("State With Arguments")) -> ("State with Arguments"=w184:string)  [unwired: 4 in]
        n72 = call <vilib>:"Build State String with Arguments__JKI_lib_State_Machine.vi"("Arguments (\"\")"=w173, "State"=w175) -> ("State with Arguments"=w172:string)  [unwired: 4 in]
        n73 = call <vilib>:"Build State String with Arguments__JKI_lib_State_Machine.vi"("Arguments (\"\")"=w181, "State"=w179) -> ("State with Arguments"=w186:string)  [unwired: 4 in]
        n74 = call <vilib>:"Build State String with Arguments__JKI_lib_State_Machine.vi"("Arguments (\"\")"=w182, "State"=w177) -> ("State with Arguments"=w185:string)  [unwired: 4 in]
        n75 = Build Array(w186, w185, w184) -> (w183:string[])
        n76 = call "CSM - Compact Multiple States.vi"("Multiple States"=w183) -> ("States"=w188:string)  [unwired: 9 in]
        n77 = call <vilib>:"Add State(s) to Queue__JKI_lib_State_Machine.vi"("State(s) in Front (\"\")"=w188, "State(s) in (\"\")"=w189, "State(s) at Back (\"\")"=w172) -> ("States Out"=w190:string)  [unwired: 12 in]
      }
      frame "Macro: TestMacroWithNonLocalSubMessages" {
        w205 = "PostMessage1" ("State With Arguments")
        w206 = "SubMessage2" ("State With Arguments")
        w208 = "SubMessage1" ("State With Arguments")
        n78 = Match Pattern(string=w201, regular expression="+") -> (before substring=w193:string, after substring=w192:string)  [unwired: 1 in, 2 out]
        n79 = call "uuid.vi"() -> ("UUID"=w204:string)  [unwired: 11 in]
        n80 = call "uuid.vi"() -> ("UUID"=w207:string)  [unwired: 11 in]
        n81 = call "uuid.vi"() -> ("UUID"=w209:string)  [unwired: 11 in]
        n82 = Concatenate Strings(w205, w204) -> (w203:string)
        n83 = Concatenate Strings(w208, w209) -> (w210:string)
        n84 = Concatenate Strings(w206, w207) -> (w211:string)
        n85 = call <vilib>:"Build State String with Arguments__JKI_lib_State_Machine.vi"("Arguments (\"\")"=w203, "State"=w205) -> ("State with Arguments"=w202:string)  [unwired: 4 in]
        n86 = call-poly "Build Message with Arguments++.vi"("State With Arguments"="SubMessage1", "Target Module (\"\")"=w192) -> ("CSM Message String"=w197:string)  [unwired: 13 in]
        n87 = call-poly "Build Message with Arguments++.vi"("State With Arguments"="SubMessage2", "Target Module (\"\")"=w192) -> ("CSM Message String"=w196:string)  [unwired: 13 in]
        n88 = call <vilib>:"Build State String with Arguments__JKI_lib_State_Machine.vi"("Arguments (\"\")"=w193, "State"="SubMessage3" ("State With Arguments")) -> ("State with Arguments"=w213:string)  [unwired: 4 in]
        n89 = call-poly "Build Message with Arguments++.vi"("State With Arguments"="Message", "Target Module (\"\")"=w192) -> ("CSM Message String"=w198:string)  [unwired: 13 in]
        n90 = call <vilib>:"Build State String with Arguments__JKI_lib_State_Machine.vi"("Arguments (\"\")"=w210, "State"=w208) -> ("State with Arguments"=w215:string)  [unwired: 4 in]
        n91 = call <vilib>:"Build State String with Arguments__JKI_lib_State_Machine.vi"("Arguments (\"\")"=w211, "State"=w206) -> ("State with Arguments"=w214:string)  [unwired: 4 in]
        n92 = Build Array(w215, w214, w213, w198, w197, w196) -> (w212:string[])
        n93 = call "CSM - Compact Multiple States.vi"("Multiple States"=w212) -> ("States"=w217:string)  [unwired: 9 in]
        n94 = call <vilib>:"Add State(s) to Queue__JKI_lib_State_Machine.vi"("State(s) in Front (\"\")"=w217, "State(s) in (\"\")"=w218, "State(s) at Back (\"\")"=w202) -> ("States Out"=w219:string)  [unwired: 12 in]
      }
      frame "---------- API ----------" {
        # "#CSM \"Category Seperator\"\nDo not put any code in this frame."
      }
      frame "API: Test SyncMessage" {
        n95 = call "CSM - Check If Module Exists.vi"("CSM Name"=w229) -> ("error out"=w223:errorcluster, "Exist?"=w224:bool, "CSM Name (Dup)"=w228:string)  [unwired: 8 in]
        n96 = case shown="True" w224 {
          tunnel: w228 -> [_ w232]
          tunnel: [_ w231] -> w225
          frame False {
          }
          frame True {
            n97 = call "uuid.vi"() -> ("UUID"=w233:string)  [unwired: 11 in]
            n98 = call-poly "Build Message with Arguments++.vi"("State With Arguments"="Message", "Arguments (\"\")"=w233, "Target Module (\"\")"=w232) -> ("CSM Message String"=w231:string)  [unwired: 12 in]
          }
        }
        n99 = call <vilib>:"Add State(s) to Queue__JKI_lib_State_Machine.vi"("State(s) in Front (\"\")"=w225, "State(s) in (\"\")"=w226) -> ("States Out"=w227:string)  [unwired: 13 in]
      }
      frame "API: Test SyncMessage With Error" {
        n100 = call "CSM - Check If Module Exists.vi"("CSM Name"=w241) -> ("error out"=w235:errorcluster, "Exist?"=w236:bool, "CSM Name (Dup)"=w240:string)  [unwired: 8 in]
        n101 = case shown="True" w236 {
          tunnel: w240 -> [_ w244]
          tunnel: [_ w243] -> w237
          frame False {
          }
          frame True {
            n102 = call "uuid.vi"() -> ("UUID"=w245:string)  [unwired: 11 in]
            n103 = call "Build Synchronous Message with Arguments.vi"("State With Arguments"="Message With Error", "Arguments (\"\")"=w245, "Target Module (\"\")"=w244) -> ("CSM Message String"=w243:string)  [unwired: 12 in]
          }
        }
        n104 = call <vilib>:"Add State(s) to Queue__JKI_lib_State_Machine.vi"("State(s) in Front (\"\")"=w237, "State(s) in (\"\")"=w238) -> ("States Out"=w239:string)  [unwired: 13 in]
      }
      frame "API: Test SyncMessage via API" {
        n105 = call "CSM - Check If Module Exists.vi"("CSM Name"=w269) -> ("error out"=w264:errorcluster, "Exist?"=w265:bool, "CSM Name (Dup)"=w268:string)  [unwired: 8 in]
        n106 = case shown="True" w265 {
          tunnel: w268 -> [_ w278]
          tunnel: [_ w277] -> w252
          tunnel: w254 -> [_ w276]
          tunnel: [_ w275] -> w261
          tunnel: [_ w274] -> w250
          tunnel: [_ w273] -> w257
          tunnel: [_ w272] -> w260
          frame False {
          }
          frame True {
            w275 = "Message" ("State With Arguments")
            n107 = call "uuid.vi"() -> ("UUID"=w273:string)  [unwired: 11 in]
            n108 = call "CSM - Wait and Send Message for Reply.vi"("State"=w275, "Current Module (\"\" to Generate an ID)"=w276, "Arguments (\"\")"=w273, "Target Module"=w278) -> ("Response"=w272:string, "Source CSM"=w274:string, "error out"=w277:errorcluster)  [unwired: 9 in]
          }
        }
        n109 = call "Strip CSM name.vi"("CSM name"=w254) -> ("error out"=w251:errorcluster, "CSM name core"=w253:string)  [unwired: 7 in, 2 out]
        n110 = call "Strip CSM name.vi"("CSM name"=w250) -> ("error out"=w247:errorcluster, "CSM name core"=w249:string)  [unwired: 7 in, 2 out]
        n111 = Bundle By Name(cluster=T1 {"Arguments"="", "Response"="", "error"={"status"=FALSE, "code"=0, "source"=""}}, "Arguments"=w257, "Response"=w260, "error"=w252) -> (w255:T1)
        n112 = Concatenate Strings(w249, ":" ("string"), w261) -> (w259:string)
        n113 = Merge Errors(w251, w247) -> (w248:errorcluster)
        n114 = call "CSM - Set Module Attribute.vi"("CSM Name"=w253, "Attribute"=w259, "Value"=w255, "Error In"=w248) -> ("error out"=w258:errorcluster)  [unwired: 8 in, 3 out]
        n115 = disable-structure shown="Enabled" {
          disable-tunnel: w255 -> [w271 _]
          frame Enabled {
            n116 = global write "Global-TestcaseCSM.vi" "response"(w271) -> ()
          }
          frame Disabled {
          }
        }
        n117 = call <vilib>:"Add State(s) to Queue__JKI_lib_State_Machine.vi"("State(s) in (\"\")"=w266) -> ("States Out"=w267:string)  [unwired: 14 in]
        n118 = Merge Errors(w258, w252, w264) -> (w263:errorcluster)
      }
      frame "API: Test SyncMessage With Error via API" {
        n119 = call "CSM - Check If Module Exists.vi"("CSM Name"=w301) -> ("error out"=w296:errorcluster, "Exist?"=w297:bool, "CSM Name (Dup)"=w300:string)  [unwired: 8 in]
        n120 = case shown="True" w297 {
          tunnel: w300 -> [_ w310]
          tunnel: [_ w309] -> w283
          tunnel: w286 -> [_ w308]
          tunnel: [_ w307] -> w293
          tunnel: [_ w306] -> w282
          tunnel: [_ w305] -> w289
          tunnel: [_ w304] -> w292
          frame False {
          }
          frame True {
            w307 = "Message With Error" ("State With Arguments")
            n121 = call "uuid.vi"() -> ("UUID"=w305:string)  [unwired: 11 in]
            n122 = call "CSM - Wait and Send Message for Reply.vi"("State"=w307, "Current Module (\"\" to Generate an ID)"=w308, "Arguments (\"\")"=w305, "Target Module"=w310) -> ("Response"=w304:string, "Source CSM"=w306:string, "error out"=w309:errorcluster)  [unwired: 9 in]
          }
        }
        n123 = call "Strip CSM name.vi"("CSM name"=w282) -> ("error out"=w279:errorcluster, "CSM name core"=w281:string)  [unwired: 7 in, 2 out]
        n124 = Bundle By Name(cluster=T1 {"Arguments"="", "Response"="", "error"={"status"=FALSE, "code"=0, "source"=""}}, "Arguments"=w289, "Response"=w292, "error"=w283) -> (w288:T1)
        n125 = call "Strip CSM name.vi"("CSM name"=w286) -> ("error out"=w284:errorcluster, "CSM name core"=w285:string)  [unwired: 7 in, 2 out]
        n126 = Concatenate Strings(w281, ":" ("string"), w293) -> (w291:string)
        n127 = Merge Errors(w284, w279) -> (w280:errorcluster)
        n128 = disable-structure shown="Enabled" {
          disable-tunnel: w288 -> [w303 _]
          frame Enabled {
            n129 = global write "Global-TestcaseCSM.vi" "response"(w303) -> ()
          }
          frame Disabled {
          }
        }
        n130 = call "CSM - Set Module Attribute.vi"("CSM Name"=w285, "Attribute"=w291, "Value"=w288, "Error In"=w280) -> ("error out"=w290:errorcluster)  [unwired: 8 in, 3 out]
        n131 = call <vilib>:"Add State(s) to Queue__JKI_lib_State_Machine.vi"("State(s) in (\"\")"=w298) -> ("States Out"=w299:string)  [unwired: 14 in]
        n132 = Merge Errors(w290, w283, w296) -> (w295:errorcluster)
      }
      frame "API: Test AsyncMessageWithReply" {
        n133 = call "CSM - Check If Module Exists.vi"("CSM Name"=w317) -> ("error out"=w311:errorcluster, "Exist?"=w312:bool, "CSM Name (Dup)"=w316:string)  [unwired: 8 in]
        n134 = case shown="True" w312 {
          tunnel: w316 -> [_ w320]
          tunnel: [_ w319] -> w313
          frame False {
          }
          frame True {
            n135 = call "uuid.vi"() -> ("UUID"=w321:string)  [unwired: 11 in]
            n136 = call-poly "Build Message with Arguments++.vi"("State With Arguments"="Message", "Arguments (\"\")"=w321, "Target Module (\"\")"=w320) -> ("CSM Message String"=w319:string)  [unwired: 12 in]
          }
        }
        n137 = call <vilib>:"Add State(s) to Queue__JKI_lib_State_Machine.vi"("State(s) in Front (\"\")"=w313, "State(s) in (\"\")"=w314) -> ("States Out"=w315:string)  [unwired: 13 in]
      }
      frame "API: Test AsyncMessageWithReply With Error" {
        n138 = call "CSM - Check If Module Exists.vi"("CSM Name"=w329) -> ("error out"=w323:errorcluster, "Exist?"=w324:bool, "CSM Name (Dup)"=w328:string)  [unwired: 8 in]
        n139 = case shown="True" w324 {
          tunnel: w328 -> [_ w333]
          tunnel: [_ w331] -> w325
          frame False {
          }
          frame True {
            n140 = call "uuid.vi"() -> ("UUID"=w332:string)  [unwired: 11 in]
            n141 = call-poly "Build Message with Arguments++.vi"("State With Arguments"="Message With Error", "Arguments (\"\")"=w332, "Target Module (\"\")"=w333) -> ("CSM Message String"=w331:string)  [unwired: 12 in]
          }
        }
        n142 = call <vilib>:"Add State(s) to Queue__JKI_lib_State_Machine.vi"("State(s) in Front (\"\")"=w325, "State(s) in (\"\")"=w326) -> ("States Out"=w327:string)  [unwired: 13 in]
      }
      frame "API: Test AsyncMessageWithoutReply" {
        n143 = call "CSM - Check If Module Exists.vi"("CSM Name"=w341) -> ("error out"=w335:errorcluster, "Exist?"=w336:bool, "CSM Name (Dup)"=w340:string)  [unwired: 8 in]
        n144 = case shown="True" w336 {
          tunnel: w340 -> [_ w346]
          tunnel: [_ w344] -> w337
          frame False {
          }
          frame True {
            n145 = call-poly "Build Message with Arguments++.vi"("State With Arguments"="AsyncMessageWithoutReply", "Arguments (\"\")"="123456789" ("Arguments (\"\")"), "Target Module (\"\")"=w346) -> ("CSM Message String"=w344:string)  [unwired: 12 in]
          }
        }
        n146 = call <vilib>:"Add State(s) to Queue__JKI_lib_State_Machine.vi"("State(s) in Front (\"\")"=w337, "State(s) in (\"\")"=w338) -> ("States Out"=w339:string)  [unwired: 13 in]
      }
      frame "API: Test AsyncMessageWithoutReply via API" {
        n147 = call "CSM - Check If Module Exists.vi"("CSM Name"=w355) -> ("error out"=w350:errorcluster, "Exist?"=w351:bool, "CSM Name (Dup)"=w354:string)  [unwired: 8 in]
        n148 = case shown="True" w351 {
          tunnel: w354 -> [_ w358]
          tunnel: w349 -> [_ w361]
          tunnel: [_ w357] -> w347
          frame False {
          }
          frame True {
            n149 = call "CSM - Wait and Post Message.vi"("State"="AsyncMessageWithoutReply" ("State With Arguments"), "Current Module (\"\" to Generate an ID)"=w361, "Arguments (\"\")"="123456789" ("Arguments (\"\")"), "Target Module"=w358) -> ("error out"=w357:errorcluster)  [unwired: 11 in]
          }
        }
        n150 = call <vilib>:"Add State(s) to Queue__JKI_lib_State_Machine.vi"("State(s) in (\"\")"=w352) -> ("States Out"=w353:string)  [unwired: 14 in]
        n151 = Merge Errors(w347, w350) -> (w348:errorcluster)
      }
      frame "API: Test Argument" {
        n152 = call "uuid.vi"() -> ("UUID"=w367:string)  [unwired: 11 in]
        n153 = call "CSM - Convert HexStr to Data.vi"("HEX String"=w371) -> ("Variant"=w369:variant, "error out"=w370:errorcluster)  [unwired: 7 in]
        n154 = Bundle("", "UUID"=w367) -> (w365:cluster{string, "UUID":string})  [unwired: 1 in]
        n155 = Variant To Data(error in=w370, type=w365, Variant=w369) -> (data=w364:cluster{string, "UUID":string}, error out=w368:errorcluster)
        n156 = Unbundle(w364) -> (w363:string, "UUID"=w362:string)
        n157 = call "CSM - Check If Module Exists.vi"("Error In"=w368, "CSM Name"=w363) -> ("error out"=w372:errorcluster, "Exist?"=w373:bool, "CSM Name (Dup)"=w377:string)  [unwired: 7 in]
        n158 = case shown="True" w373 {
          tunnel: w377 -> [_ w381]
          tunnel: [_ w380] -> w374
          tunnel: w362 -> [_ w379]
          frame False {
          }
          frame True {
            n159 = call "Build Synchronous Message with Arguments.vi"("State With Arguments"="ArgumentTest", "Arguments (\"\")"=w379, "Target Module (\"\")"=w381) -> ("CSM Message String"=w380:string)  [unwired: 12 in]
          }
        }
        n160 = call <vilib>:"Add State(s) to Queue__JKI_lib_State_Machine.vi"("State(s) in Front (\"\")"=w374, "State(s) in (\"\")"=w375) -> ("States Out"=w376:string)  [unwired: 13 in]
      }
      frame "API: Test Argument Only For Chain4", "API: Test Argument Only For Chain4And5", "API: Test Argument Only For Chain4And5And6", "API: Test Argument Only For Chain4And6", "API: Test Argument Only For Chain5", "API: Test Argument Only For Chain5And6", "API: Test Argument Only For Chain6" {
        n161 = call "uuid.vi"() -> ("UUID"=w401:string)  [unwired: 11 in]
        n162 = call "CSM - Convert HexStr to Data.vi"("HEX String"=w405) -> ("Variant"=w403:variant, "error out"=w404:errorcluster)  [unwired: 7 in]
        n163 = Match Pattern(string=w389, regular expression="Chain") -> (after substring=w384:string, offset past match=w387:i32)  [unwired: 1 in, 2 out]
        n164 = Bundle("", "UUID"=w401) -> (w399:cluster{string, "UUID":string})  [unwired: 1 in]
        n165 = Variant To Data(error in=w404, type=w399, Variant=w403) -> (data=w398:cluster{string, "UUID":string}, error out=w402:errorcluster)
        n166 = Not Equal?(x=w387, y=-1) -> (x != y?=w385:bool)
        n167 = call "CSM - Resolve Node Module.vi"("Node Name"=w395) -> ("CSM Module Name"=w394:string)  [unwired: 10 in]
        n168 = case shown="True" w385 {
          tunnel: w384 -> [_ w411]
          tunnel: [_ w411] -> w383
          frame False {
          }
          frame True {
          }
        }
        n169 = Unbundle(w398) -> (w397:string, "UUID"=w396:string)
        n170 = call "CSM - Check If Module Exists.vi"("Error In"=w402, "CSM Name"=w397) -> ("error out"=w393:errorcluster, "Exist?"=w406:bool, "CSM Name (Dup)"=w409:string)  [unwired: 7 in]
        n171 = case shown="True" w406 {
          tunnel: w409 -> [_ w418]
          tunnel: w396 -> [_ w419]
          tunnel: [_ w417] -> w390
          tunnel: w394 -> [_ w416]
          tunnel: [_ w415] -> w392
          tunnel: w383 -> [_ w413]
          frame False {
          }
          frame True {
            n172 = Concatenate Strings("ArgumentTestOnlyForChain" ("State With Arguments"), w413) -> (w412:string)
            n173 = call "CSM - Wait and Send Message for Reply.vi"("State"=w412, "Current Module (\"\" to Generate an ID)"=w416, "Arguments (\"\")"=w419, "Target Module"=w418) -> ("Response"=w415:string, "error out"=w417:errorcluster)  [unwired: 9 in, 1 out]
          }
        }
        n174 = call <vilib>:"Add State(s) to Queue__JKI_lib_State_Machine.vi"("State(s) in (\"\")"=w407) -> ("States Out"=w408:string)  [unwired: 14 in]
        n175 = Merge Errors(w393, w390) -> (w391:errorcluster)
      }
      frame "API: Test Response With Error" {
        n176 = call "CSM - Check If Module Exists.vi"("CSM Name"=w426) -> ("error out"=w420:errorcluster, "Exist?"=w421:bool, "CSM Name (Dup)"=w425:string)  [unwired: 8 in]
        n177 = case shown="True" w421 {
          tunnel: w425 -> [_ w429]
          tunnel: [_ w428] -> w422
          frame False {
          }
          frame True {
            n178 = call "uuid.vi"() -> ("UUID"=w430:string)  [unwired: 11 in]
            n179 = call "Build Synchronous Message with Arguments.vi"("State With Arguments"="Response With Error", "Arguments (\"\")"=w430, "Target Module (\"\")"=w429) -> ("CSM Message String"=w428:string)  [unwired: 12 in]
          }
        }
        n180 = call <vilib>:"Add State(s) to Queue__JKI_lib_State_Machine.vi"("State(s) in Front (\"\")"=w422, "State(s) in (\"\")"=w423) -> ("States Out"=w424:string)  [unwired: 13 in]
      }
      frame "API: Test MacroWithSubMessages" {
        n181 = call <vilib>:"Build State String with Arguments__JKI_lib_State_Machine.vi"("Arguments (\"\")"=w433, "State"="Macro: Test MacroWithSubMessages") -> ("State with Arguments"=w432:string)  [unwired: 4 in]
        n182 = call <vilib>:"Add State(s) to Queue__JKI_lib_State_Machine.vi"("State(s) in Front (\"\")"=w432, "State(s) in (\"\")"=w436) -> ("States Out"=w435:string)  [unwired: 13 in]
      }
      frame "API: Test MacroWithSubAndPostMessages" {
        n183 = call <vilib>:"Build State String with Arguments__JKI_lib_State_Machine.vi"("Arguments (\"\")"=w440, "State"="Macro: Test MacroWithSubAndPostMessages") -> ("State with Arguments"=w439:string)  [unwired: 4 in]
        n184 = call <vilib>:"Add State(s) to Queue__JKI_lib_State_Machine.vi"("State(s) in Front (\"\")"=w439, "State(s) in (\"\")"=w443) -> ("States Out"=w442:string)  [unwired: 13 in]
      }
      frame "API: Test MacroWithNonLocalSubMessages" {
        n185 = call <vilib>:"Build State String with Arguments__JKI_lib_State_Machine.vi"("Arguments (\"\")"=w447, "State"="Macro: TestMacroWithNonLocalSubMessages") -> ("State with Arguments"=w446:string)  [unwired: 4 in]
        n186 = call <vilib>:"Add State(s) to Queue__JKI_lib_State_Machine.vi"("State(s) in Front (\"\")"=w446, "State(s) in (\"\")"=w450) -> ("States Out"=w449:string)  [unwired: 13 in]
      }
      frame "API: Test Register State" {
        n187 = call <vilib>:"Build State String with Arguments__JKI_lib_State_Machine.vi"("Arguments (\"\")"=w454, "State"="Test Status") -> ("State with Arguments"=w453:string)  [unwired: 4 in]
        n188 = call <vilib>:"Add State(s) to Queue__JKI_lib_State_Machine.vi"("State(s) in Front (\"\")"=w453, "State(s) in (\"\")"=w457) -> ("States Out"=w456:string)  [unwired: 13 in]
      }
      frame "API: Test Register State Argument Info" {
        n189 = call <vilib>:"Build State String with Arguments__JKI_lib_State_Machine.vi"("Arguments (\"\")"=w461, "State"="Register State Argument Info") -> ("State with Arguments"=w460:string)  [unwired: 4 in]
        n190 = call <vilib>:"Add State(s) to Queue__JKI_lib_State_Machine.vi"("State(s) in Front (\"\")"=w460, "State(s) in (\"\")"=w464) -> ("States Out"=w463:string)  [unwired: 13 in]
      }
      frame "API: Test Register Status" {
        n191 = call <vilib>:"Build State String with Arguments__JKI_lib_State_Machine.vi"("Arguments (\"\")"=w468, "State"="Register Status") -> ("State with Arguments"=w467:string)  [unwired: 4 in]
        n192 = call <vilib>:"Add State(s) to Queue__JKI_lib_State_Machine.vi"("State(s) in Front (\"\")"=w467, "State(s) in (\"\")"=w471) -> ("States Out"=w470:string)  [unwired: 13 in]
      }
      frame "API: Test Register Interrupt" {
        n193 = call <vilib>:"Build State String with Arguments__JKI_lib_State_Machine.vi"("Arguments (\"\")"=w475, "State"="Register Interrupt") -> ("State with Arguments"=w474:string)  [unwired: 4 in]
        n194 = call <vilib>:"Add State(s) to Queue__JKI_lib_State_Machine.vi"("State(s) in Front (\"\")"=w474, "State(s) in (\"\")"=w478) -> ("States Out"=w477:string)  [unwired: 13 in]
      }
      frame "API: Test Register Status Argument Info" {
        n195 = call <vilib>:"Build State String with Arguments__JKI_lib_State_Machine.vi"("Arguments (\"\")"=w482, "State"="Register Status Argument Info") -> ("State with Arguments"=w481:string)  [unwired: 4 in]
        n196 = call <vilib>:"Add State(s) to Queue__JKI_lib_State_Machine.vi"("State(s) in Front (\"\")"=w481, "State(s) in (\"\")"=w485) -> ("States Out"=w484:string)  [unwired: 13 in]
      }
      frame "API: Test Status A" {
        n197 = call <vilib>:"Build State String with Arguments__JKI_lib_State_Machine.vi"("Arguments (\"\")"=w489, "State"="Broadcast Status A") -> ("State with Arguments"=w490:string)  [unwired: 4 in]
        n198 = call <vilib>:"Add State(s) to Queue__JKI_lib_State_Machine.vi"("State(s) in Front (\"\")"=w490, "State(s) in (\"\")"=w492) -> ("States Out"=w491:string)  [unwired: 13 in]
      }
      frame "API: Test State A" {
        n199 = call <vilib>:"Build State String with Arguments__JKI_lib_State_Machine.vi"("Arguments (\"\")"=w496, "State"="State A") -> ("State with Arguments"=w497:string)  [unwired: 4 in]
        n200 = call <vilib>:"Add State(s) to Queue__JKI_lib_State_Machine.vi"("State(s) in Front (\"\")"=w497, "State(s) in (\"\")"=w499) -> ("States Out"=w498:string)  [unwired: 13 in]
      }
      frame "API: Test State B" {
        n201 = call <vilib>:"Build State String with Arguments__JKI_lib_State_Machine.vi"("Arguments (\"\")"=w503, "State"="State B") -> ("State with Arguments"=w504:string)  [unwired: 4 in]
        n202 = call <vilib>:"Add State(s) to Queue__JKI_lib_State_Machine.vi"("State(s) in Front (\"\")"=w504, "State(s) in (\"\")"=w506) -> ("States Out"=w505:string)  [unwired: 13 in]
      }
      frame "API: Test Status B" {
        n203 = call <vilib>:"Build State String with Arguments__JKI_lib_State_Machine.vi"("Arguments (\"\")"=w510, "State"="Broadcast Status B") -> ("State with Arguments"=w511:string)  [unwired: 4 in]
        n204 = call <vilib>:"Add State(s) to Queue__JKI_lib_State_Machine.vi"("State(s) in Front (\"\")"=w511, "State(s) in (\"\")"=w513) -> ("States Out"=w512:string)  [unwired: 13 in]
      }
      frame "API: Local Registration" {
        # "Test Status @ From >> Handler Message @ To -><register>"
        n205 = call "Strip CSM name.vi"("CSM name"=w521) -> ("error out"=w519:errorcluster, "CSM name core"=w516:string)  [unwired: 7 in, 2 out]
        n206 = call-poly "Build Message with Arguments++.vi"("Target CSM"=w517, "Source CSM (* as Default)"=w516, "Status"="Test Status", "API (If \"\", Same As \"Status\")"="Handler Message") -> ("CSM Message String"=w518:string)  [unwired: 11 in]
        n207 = call <vilib>:"Add State(s) to Queue__JKI_lib_State_Machine.vi"("State(s) in Front (\"\")"=w518, "State(s) in (\"\")"=w525) -> ("States Out"=w524:string)  [unwired: 13 in]
      }
      frame "API: Local Registration II" {
        # "Test Status @ From >> Handler Message -><register>"
        n208 = call "Strip CSM name.vi"("CSM name"=w530) -> ("error out"=w528:errorcluster, "CSM name core"=w526:string)  [unwired: 7 in, 2 out]
        n209 = call-poly "Build Message with Arguments++.vi"("Source CSM (* as Default)"=w526, "Status"="Test Status", "API (If \"\", Same As \"Status\")"="Handler Message") -> ("CSM Message String"=w527:string)  [unwired: 12 in]
        n210 = call <vilib>:"Add State(s) to Queue__JKI_lib_State_Machine.vi"("State(s) in Front (\"\")"=w527, "State(s) in (\"\")"=w534) -> ("States Out"=w533:string)  [unwired: 13 in]
      }
      frame "API: Local Unregistration" {
        # "Test Status @ From >> Handler Message @ To -><unregister>"
        n211 = call "Strip CSM name.vi"("CSM name"=w540) -> ("error out"=w538:errorcluster, "CSM name core"=w535:string)  [unwired: 7 in, 2 out]
        n212 = call-poly "Build Message with Arguments++.vi"("Target CSM"=w536, "Source CSM (* as Default)"=w535, "Status"="Test Status", "API (If \"\", Same As \"Status\")"="Handler Message") -> ("CSM Message String"=w537:string)  [unwired: 11 in]
        n213 = call <vilib>:"Add State(s) to Queue__JKI_lib_State_Machine.vi"("State(s) in Front (\"\")"=w537, "State(s) in (\"\")"=w544) -> ("States Out"=w543:string)  [unwired: 13 in]
      }
      frame "API: Local Registration via API" {
        # "Test Status @ From >> Handler Message @ To -><register>"
        n214 = call "Strip CSM name.vi"("CSM name"=w551) -> ("error out"=w550:errorcluster, "CSM name core"=w546:string)  [unwired: 7 in, 2 out]
        n215 = call "CSM - Register Broadcast.vi"("CSM Name(Empty for Broadcast Event)"=w545, "Source CSM Name (* as Default)"=w546, "Trigger"="Test Status", "API (If \"\", Same as Trigger)"="Handler Message", "Error In"=w550) -> ("error out"=w549:errorcluster)  [unwired: 9 in, 1 out]
        n216 = call <vilib>:"Add State(s) to Queue__JKI_lib_State_Machine.vi"("State(s) in (\"\")"=w554) -> ("States Out"=w553:string)  [unwired: 14 in]
      }
      frame "API: Local Unregistration via API" {
        # "Test Status @ From >> Handler Message @ To -><unregister>"
        n217 = call "Strip CSM name.vi"("CSM name"=w561) -> ("error out"=w560:errorcluster, "CSM name core"=w556:string)  [unwired: 7 in, 2 out]
        n218 = call "CSM - Unregister Broadcast.vi"("CSM Name(Empty for Broadcast Event)"=w555, "Source CSM Name (* as Default)"=w556, "Trigger"="Test Status", "API (\"*\" as Default)"="Handler Message", "Error In"=w560) -> ("error out"=w559:errorcluster)  [unwired: 9 in, 1 out]
        n219 = call <vilib>:"Add State(s) to Queue__JKI_lib_State_Machine.vi"("State(s) in (\"\")"=w564) -> ("States Out"=w563:string)  [unwired: 14 in]
      }
      frame "API: API2" {
        # "#CSM API Example\nCopy/Rename this case for your own API"
        # "unpack Hex String  to Variant\nif complex parameter is needed."
        n220 = call "CSM - Convert HexStr to Data.vi"("HEX String"=w566) -> ()  [unwired: 7 in, 2 out]
        n221 = disable-structure shown="Enabled" {
          disable-tunnel: [w569 "API2 Response"] -> w565
          frame Disabled {
            # "pack variant to hexstr \nif complex response is needed."
            # "complex Response"
            n222 = call "CSM - Convert Data to HexStr.vi"() -> ("HEX String (0-9,A-F)"=w569:string)  [unwired: 9 in]
          }
          frame Enabled {
          }
        }
      }
      frame "---------- Action ----------" {
        # "#CSM \"Category Seperator\"\nDo not put any code in this frame."
        n223 = call <vilib>:"Add State(s) to Queue__JKI_lib_State_Machine.vi"("State(s) in (\"\")"=w573) -> ("States Out"=w572:string)  [unwired: 14 in]
      }
      frame "Action: action1" {
        # "#CSM \"Internal State\"\nThis category is used for holding internal states"
        n224 = call <vilib>:"Add State(s) to Queue__JKI_lib_State_Machine.vi"("State(s) in (\"\")"=w576) -> ("States Out"=w575:string)  [unwired: 14 in]
      }
      frame "Test Status" {
        n225 = call <vilib>:"Add State(s) to Queue__JKI_lib_State_Machine.vi"("State(s) in (\"\")"=w580) -> ("States Out"=w579:string)  [unwired: 14 in]
      }
      frame "Register State Argument Info" {
        n226 = call "Strip CSM name.vi"("CSM name"=w584) -> ("error out"=w583:errorcluster, "CSM name core"=w585:string)  [unwired: 7 in, 2 out]
        n227 = Concatenate Strings(w581, "+", w585) -> (w582:string)
        n228 = call <vilib>:"Add State(s) to Queue__JKI_lib_State_Machine.vi"("State(s) in (\"\")"=w587) -> ("States Out"=w589:string)  [unwired: 14 in]
      }
      frame "Register Status" {
        n229 = call <vilib>:"Build State String with Arguments__JKI_lib_State_Machine.vi"("Arguments (\"\")"=w590, "State"="Test Status") -> ("State with Arguments"=w592:string)  [unwired: 4 in]
        n230 = call "CSM - Broadcast Status Change.vi"("Status With Arguments"=w592, "State Queue"=w594) -> ("Remaining States"=w591:string)  [unwired: 13 in]
      }
      frame "Register Interrupt" {
        n231 = call-poly "Build Message with Arguments++.vi"("State With Arguments"="Test Interrupt", "Arguments (\"\")"=w599) -> ("CSM Message String"=w598:string)  [unwired: 13 in]
        n232 = call <vilib>:"Add State(s) to Queue__JKI_lib_State_Machine.vi"("State(s) in Front (\"\")"=w598, "State(s) in (\"\")"=w597) -> ("States Out"=w596:string)  [unwired: 13 in]
      }
      frame "Register Status Argument Info" {
        w607 = "Test Status Argument Info"
        n233 = call "Strip CSM name.vi"("CSM name"=w605) -> ("error out"=w603:errorcluster, "CSM name core"=w604:string)  [unwired: 7 in, 2 out]
        n234 = Concatenate Strings(w607, "+", w604) -> (w602:string)
        n235 = call <vilib>:"Build State String with Arguments__JKI_lib_State_Machine.vi"("Arguments (\"\")"=w602, "State"=w607) -> ("State with Arguments"=w609:string)  [unwired: 4 in]
        n236 = call "CSM - Broadcast Status Change.vi"("Status With Arguments"=w609, "State Queue"=w610) -> ("Remaining States"=w608:string)  [unwired: 13 in]
      }
      frame "Broadcast Status A" {
        n237 = call <vilib>:"Build State String with Arguments__JKI_lib_State_Machine.vi"("Arguments (\"\")"=w612, "State"="Status A") -> ("State with Arguments"=w614:string)  [unwired: 4 in]
        n238 = call "CSM - Broadcast Status Change.vi"("Status With Arguments"=w614, "State Queue"=w616) -> ("Remaining States"=w613:string)  [unwired: 13 in]
      }
      frame "Broadcast Status B" {
        n239 = call <vilib>:"Build State String with Arguments__JKI_lib_State_Machine.vi"("Arguments (\"\")"=w618, "State"="Status B") -> ("State with Arguments"=w620:string)  [unwired: 4 in]
        n240 = call "CSM - Broadcast Status Change.vi"("Status With Arguments"=w620, "State Queue"=w622) -> ("Remaining States"=w619:string)  [unwired: 13 in]
      }
      frame "State A" {
        n241 = call <vilib>:"Add State(s) to Queue__JKI_lib_State_Machine.vi"("State(s) in (\"\")"=w626) -> ("States Out"=w625:string)  [unwired: 14 in]
      }
      frame "State B" {
        n242 = call <vilib>:"Add State(s) to Queue__JKI_lib_State_Machine.vi"("State(s) in (\"\")"=w631) -> ("States Out"=w630:string)  [unwired: 14 in]
      }
      frame "Message" {
      }
      frame "SubMessage1" {
      }
      frame "SubMessage2" {
      }
      frame "SubMessage3" {
        n243 = call "Strip CSM name.vi"("CSM name"=w652) -> ("error out"=w650:errorcluster, "CSM name core"=w651:string)  [unwired: 7 in, 2 out]
        n244 = call "CSM - Set Module Attribute.vi"("CSM Name"=w651, "Attribute"=w649, "Value"=w648, "Error In"=w650) -> ("error out"=w646:errorcluster)  [unwired: 8 in, 3 out]
        n245 = Merge Errors(w646, w655) -> (w647:errorcluster)
      }
      frame "PostMessage1" {
      }
      frame "Message With Error" {
        n246 = Merge Errors(errorcluster {"status"=TRUE, "code"=1234567898, "source"="Simulated Error\nwill be sent to Response case"} ("error out"), w661) -> (w660:errorcluster)
      }
      frame "Response With Error" {
        n247 = Merge Errors(errorcluster {"status"=TRUE, "code"=1234567898, "source"="Simulated Error"} ("error out"), w667) -> (w666:errorcluster)
      }
      frame "ArgumentTest" {
        n248 = call "Strip CSM name.vi"("CSM name"=w678) -> ("error out"=w675:errorcluster, "CSM name core"=w677:string)  [unwired: 7 in, 2 out]
        n249 = call "CSM - Set Module Attribute.vi"("CSM Name"=w677, "Attribute"=w674, "Value"=w676, "Error In"=w675) -> ("error out"=w672:errorcluster)  [unwired: 8 in, 3 out]
        n250 = Merge Errors(w672, w681) -> (w673:errorcluster)
      }
      frame "ArgumentTestOnlyForChain4", "ArgumentTestOnlyForChain4And5", "ArgumentTestOnlyForChain4And5And6", "ArgumentTestOnlyForChain4And6", "ArgumentTestOnlyForChain5", "ArgumentTestOnlyForChain5And6", "ArgumentTestOnlyForChain6" {
        n251 = call "Strip CSM name.vi"("CSM name"=w682) -> ("error out"=w687:errorcluster, "CSM name core"=w688:string)  [unwired: 7 in, 2 out]
        n252 = call "CSM - Set Module Attribute.vi"("CSM Name"=w688, "Attribute"=w682, "Value"=w682, "Error In"=w687) -> ("error out"=w684:errorcluster)  [unwired: 8 in, 3 out]
        n253 = Merge Errors(w684, w690) -> (w686:errorcluster)
      }
      frame "AsyncMessageWithoutReply" {
        # "123456789 string constant"
        n254 = call "Strip CSM name.vi"("CSM name"=w695) -> ("error out"=w693:errorcluster, "CSM name core"=w694:string)  [unwired: 7 in, 2 out]
        n255 = call "CSM - Set Module Attribute.vi"("CSM Name"=w694, "Attribute"=w696, "Value"=w697, "Error In"=w693) -> ("error out"=w691:errorcluster)  [unwired: 8 in, 3 out]
        n256 = Merge Errors(w691, w700) -> (w692:errorcluster)
      }
      frame "Handler Message" {
        n257 = call "Strip CSM name.vi"("CSM name"=w707) -> ("error out"=w705:errorcluster, "CSM name core"=w706:string)  [unwired: 7 in, 2 out]
        n258 = call "CSM - Set Module Attribute.vi"("CSM Name"=w706, "Attribute"=w703, "Value"=w702, "Error In"=w705) -> ("error out"=w701:errorcluster)  [unwired: 8 in, 3 out]
        n259 = Merge Errors(w710, w701) -> (w704:errorcluster)
      }
      frame "Handler Message With Counter" {
        n260 = Unbundle By Name(w716) -> ("Counter"=w717:u32)
        n261 = Decimal String To Number(string=w714) -> (number=w711:i32)  [unwired: 2 in, 1 out]
        n262 = Increment(x=w717) -> (x+1=w712:u32)
        n263 = Bundle By Name(cluster=w716, "Counter"=w712) -> (w715:T6)
        n264 = Equal?(x=w712, y=w711) -> (x = y?=w713:bool)
        n265 = call "Strip CSM name.vi"("CSM name"=w723) -> ("error out"=w721:errorcluster, "CSM name core"=w722:string)  [unwired: 7 in, 2 out]
        n266 = case shown="True" w713 {
          tunnel: w722 -> [_ w731]
          tunnel: w721 -> [w726 w730]
          tunnel: w719 -> [_ w729]
          tunnel: [w726 w728] -> w718
          tunnel: w712 -> [_ w727]
          frame False {
          }
          frame True {
            n267 = call "CSM - Set Module Attribute.vi"("CSM Name"=w731, "Attribute"=w729, "Value"=w727, "Error In"=w730) -> ("error out"=w728:errorcluster)  [unwired: 8 in, 3 out]
          }
        }
        n268 = Merge Errors(w725, w718) -> (w720:errorcluster)
      }
      frame "Reset Counter" {
        # "#CSM \"Internal State\"\nThis category is used for holding internal states"
        n269 = Bundle By Name(cluster=w734, "Counter"=u32 0) -> (w732:T6)
        n270 = call <vilib>:"Add State(s) to Queue__JKI_lib_State_Machine.vi"("State(s) in (\"\")"=w736) -> ("States Out"=w735:string)  [unwired: 14 in]
      }
    }
  }
